vi "SendActionEventSync.vi"(8 "error in (no error)":errorcluster, 9 "Variant":variant, 10 "Action":T1, 11 "WindowFrame in":refnum<class "WindowFrame.lvclass">) -> (0 "error out":errorcluster, 3 "WindowFrame out":refnum<class "WindowFrame.lvclass">)   [LabVIEW 2021, in "WindowFrame.lvlib" / "WindowFrame.lvclass"]
uses:
  WindowFrame.lvclass
  Action.ctl
  C:/GitHub/ClassUtilities/src/ClassByRef/ClassByRef.lvclass
  ActionData.ctl
  ClassUtilities/src/ClassByRef/ClassByRef.lvclass/ClassByRef.ctl
  ClassUtilities/src/ClassByRef/SetNotifier.vi
  <vilib>/Utility/error.llb/Clear Errors.vi
  ClassUtilities/src/ClassByRef/GetNotifier.vi
  ClassUtilities/src/ClassByRef/SetNotifier.vi/6a7be9d6-cac5-4ac9-b7fd-da113b1d2d73.vi
  ClassUtilities/src/ClassByRef/GetNotifier.vi/815770e3-f244-4544-877a-43bf45f14863.vi
  ClassUtilities/src/ClassByRef/GetRef.vi
  <vilib>/Utility/error.llb/Error Cluster From Error Code.vi
  GetEventActionRef.vi
  ClassUtilities/src/ClassByRef/ClassByRef.lvclass
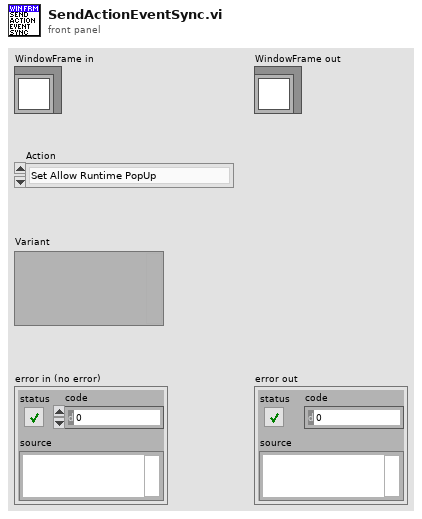
[diagram p1: front panel]
types:
  T1 = typedef "WindowFrame.lvlib/WindowFrame.lvclass/Action.ctl" = enum16{"Set Allow Runtime PopUp", "Set Behavior", "Set Closable", "Set Custom Title", "Set Highlight Return Button", "Set Is Frontmost", "Set Minimizable", "Set Minimum Size", "Set Monitor", "Set Resizable", "Set Panel Bounds", "Set Run VI Transparently", "Set Show Menu Bar", "Set State", "Set Title", "Set Title Bar Colors", "Set Title Bar Visible", "Set Transparancy", "Set Window Bounds", "Get Allow Runtime PopUp", "Get Behavior", "Get Closable", "Get Custom Title", "Get Highlight Return Button", "Get Is Frontmost", "Get Minimizable", "Get Minimum Size", "Get Monitor", "Get Panel Bounds", "Get Resizable", "Get Run VI Transparently", "Get Show Menu Bar", "Get State", "Get Title", "Get Title Bar Colors", "Get Title Bar Visible", "Get Transparancy", "Get Window Bounds", "--", "Center", "Close", "Open", "Run-Time Position:Centered", "Run-Time Position:Custom", "Run-Time Position:Get Position", "Run-Time Position:Maximized", "Run-Time Position:Minimized", "Run-Time Position:Unchanged", "---", "Insert VI", "Remove VI", "Insert VI Index", "Remove VI Index", "Exit"}
  T2 = typedef "WindowFrame.lvlib/WindowFrame.lvclass/ActionData.ctl" = cluster{"Action":T1, "Variant":variant}
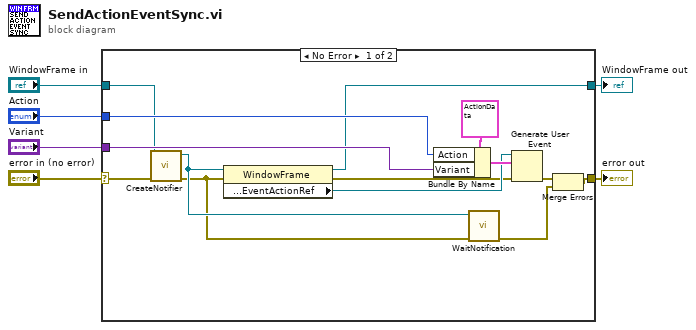
[diagram p0: block diagram]
diagram:
  n1 = case shown="No Error" "error in (no error)" {
    selector: "error in (no error)" -> [w14 w21]
    tunnel: "Action" -> [w20 _]
    tunnel: [w8 w21] -> w5
    tunnel: "WindowFrame in" -> [w11 w22]
    tunnel: [w12 w22] -> w3
    tunnel: "Variant" -> [w16 _]
    frame No Error {
      n2 = call "CreateNotifier.vi"("error in (no error)"=w14, "ByRefClass in"=w11) -> ("error out"=w9:errorcluster, "ByRefClass out"=w10:refnum<class "WindowFrame.lvclass">)  [unwired: 7 in, 1 out]
      n3 = property class="WindowFrame"(reference=w10, error in=w9) -> (reference out=w12:refnum<class "WindowFrame.lvclass">, error out=w13:errorcluster, "Private:Properties:EventActionRef"=w15:refnum<user-event>)
      n4 = Bundle By Name(cluster=T2 {"Action"=enum."Set Allow Runtime PopUp", "Variant"=variant} ("event data"), "Action"=w20, "Variant"=w16) -> (w19:T2)
      n5 = call "WaitNotification.vi"("error in (no error)"=w9, "ByRefClass in"=w10) -> ("error out"=w7:errorcluster)  [unwired: 8 in, 1 out]
      n6 = Generate User Event(user event=w15, event data cluster=w19, error in=w13) -> (error out=w18:errorcluster)  [unwired: 1 in, 1 out]
      n7 = Merge Errors(w18, w7) -> (w8:errorcluster)
    }
    frame Error {
    }
  }
  "error out" <- w5
  "WindowFrame out" <- w3
